vi "Update Last Waypoint ToolTip with Distance.vi"(8 "Error In":errorcluster) -> (0 "Error Out":errorcluster)   [LabVIEW 2014]
uses:
  C:/Robotic Systems/Products/AgFalcon/Software/Ground Station/Data/Mapping DLL/GMap.NET.WindowsForms.dll
  Data/Mapping DLL/GMap.NET.WindowsForms.dll
  Reference/SubVI/GMap DLL Refernce.vi
  Reference/SubVI/Main Map Control Refernce.vi
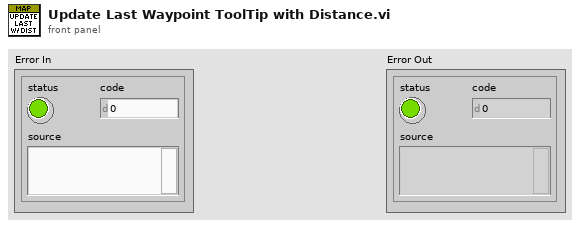
[diagram p1: front panel]
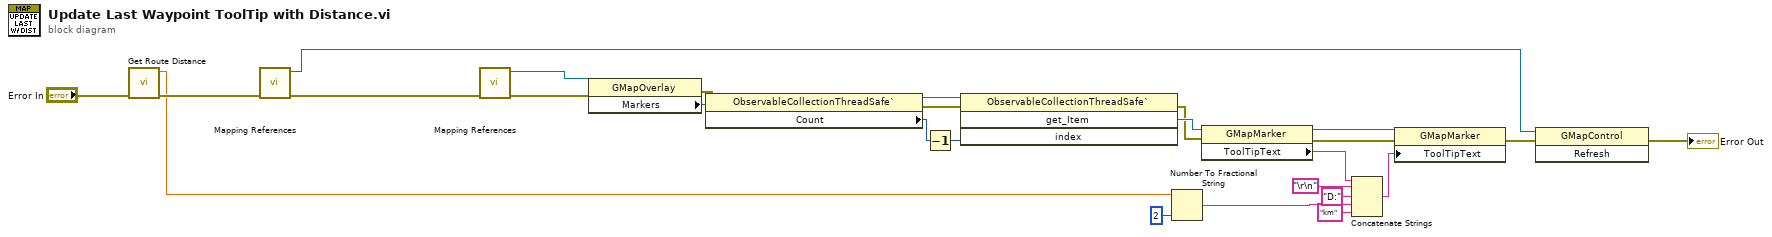
[diagram p0: block diagram]
diagram:
  n1 = call "Get Route Distance.vi"("Error In"="Error In") -> ("error out"=w22:errorcluster, "Distance"=w10:dbl)  [unwired: 9 in]
  n2 = call-poly "Mapping References.vi"("Error In"=w22) -> ("Error Out"=w24:errorcluster, "GMap DLL Reference"=w1:refnum<k24>)  [unwired: 9 in]
  n3 = call-poly "Mapping References.vi"("Error In"=w24) -> ("Error Out"=w23:errorcluster, "Main Map Reference"=w25:refnum<k24>)  [unwired: 9 in]
  n4 = property class="GMapOverlay"(reference=w25, error in=w23) -> (error out=w20:errorcluster, "Markers"=w21:refnum<k24>)  [unwired: 1 out]
  n5 = property class="ObservableCollectionThreadSafe`"(reference=w21, error in=w20) -> (reference out=w19:refnum<k24>, error out=w18:errorcluster, "Count"=w16:i32)
  n6 = Decrement(x=w16) -> (x-1=w17:i32)
  n7 = invoke class="ObservableCollectionThreadSafe`" method="get_Item"(reference=w19, error in=w18, "index"=w17) -> (error out=w14:errorcluster, "get_Item"=w15:refnum<k24>)  [unwired: 1 in, 2 out]
  n8 = Number To Fractional String(number=w10, precision (6)=i16 2) -> (F-format string=w8:string)  [unwired: 2 in]
  n9 = property class="GMapMarker"(reference=w15, error in=w14) -> (reference out=w6:refnum<k24>, error out=w5:errorcluster, "ToolTipText"=w13:string)
  n10 = Concatenate Strings(w13, "\r\n", "D:" ("string"), w8, "km" ("string")) -> (w4:string)
  n11 = property class="GMapMarker"(reference=w6, error in=w5, "ToolTipText"=w4) -> (error out=w3:errorcluster)  [unwired: 1 out]
  n12 = invoke class="GMapControl" method="Refresh"(reference=w1, error in=w3) -> (error out=→"Error Out":errorcluster)  [unwired: 1 in, 2 out]
